vi "Common_GetClassAttrubutes.vi"(1 "Path(CtrlRenumf used if Path is empty)":path, 2 "CtlRefnum":refnum<vi>, 5 "error in (no error)":errorcluster, 6 "AttributeSerachP{atternNamesToIgnore":string[](array[string])) -> (12 "LibraryName":string, 15 "attributeInfo":T1[](array[typedef]), 19 "error out":errorcluster)   [LabVIEW 2020]
uses:
  CommonVIs_AttributeInfoType.ctl
  CommonVIs_AttributeDataType.ctl
  CommonVIs_VisibilityType.ctl
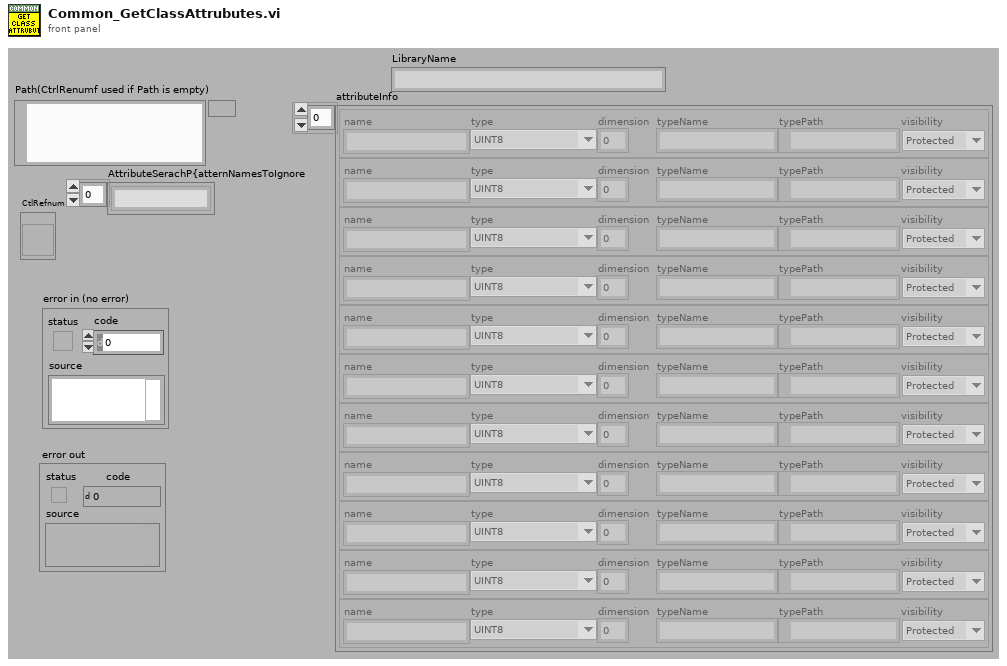
[diagram p1: front panel]
types:
  T1 = typedef "CommonVIs_AttributeInfoType.ctl" = cluster{"name":string, "type":T2, "dimension":i32, "typeName":string, "typePath":path, "visibility":T3}
  T2 = typedef "CommonVIs_AttributeDataType.ctl" = enum16{"UINT8", "INT8", "UINT16", "INT16", "UINT32", "INT32", "UINT64", "INT64", "SGL", "DBL", "EXT", "CSG", "CDB", "CXT", "TimeStamp", "STRING", "PATH", "BOOL", "ENUM", "RefNum", "VIRefNum", "LabVIEW Class", "Cluster", "Variant", "TypeDef", "Waveform", "LabVIEW Object", "Other", "void", "Set", "Map"}
  T3 = typedef "CommonVIs_VisibilityType.ctl" = enum16{"Public", "Private", "Protected"}
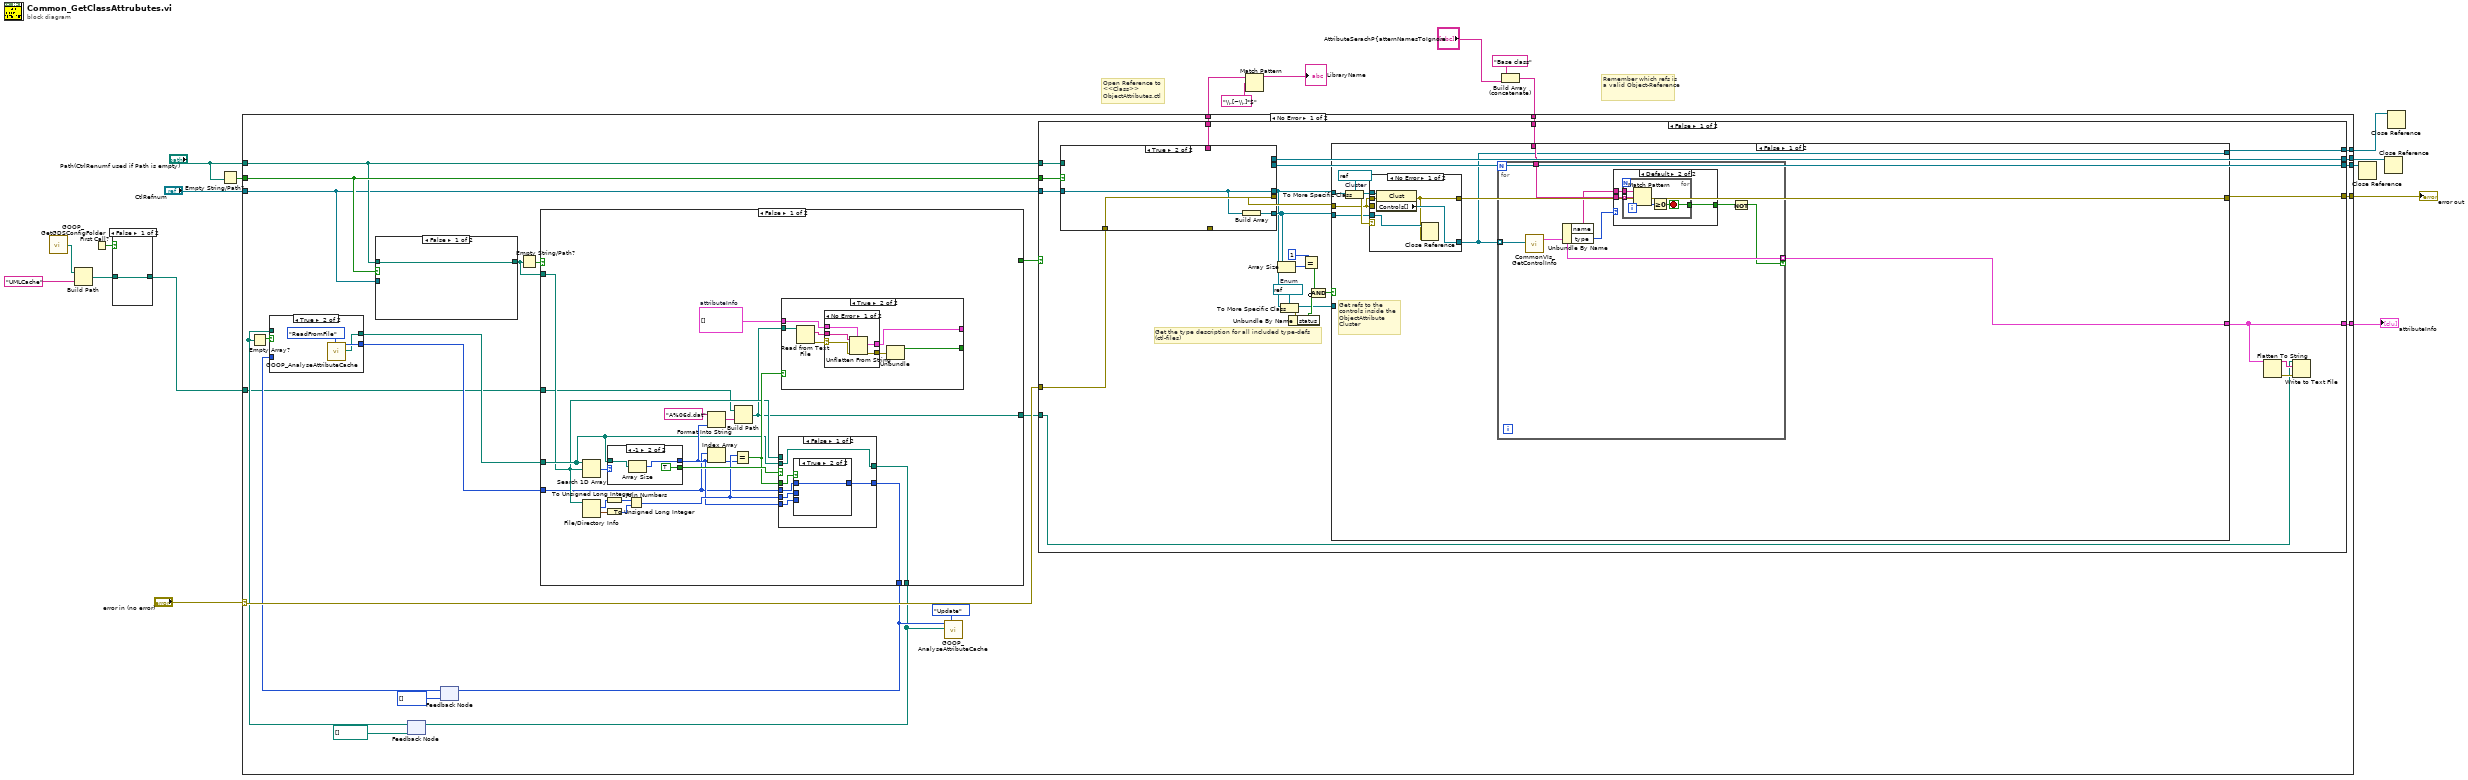
[diagram p0: block diagram]
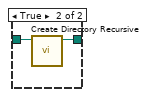
[diagram p2: hidden frame]
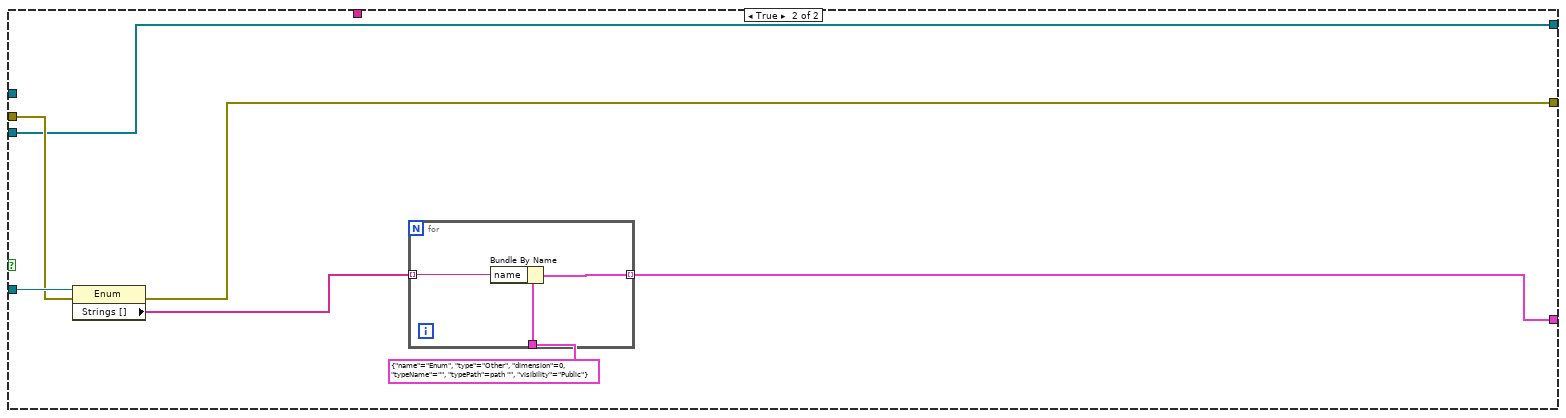
[diagram p6: hidden frame]
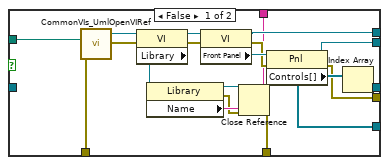
[diagram p7: hidden frame]
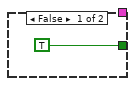
[diagram p9: hidden frame]
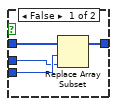
[diagram p11: hidden frame]
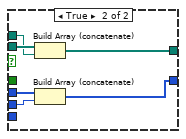
[diagram p12: hidden frame]
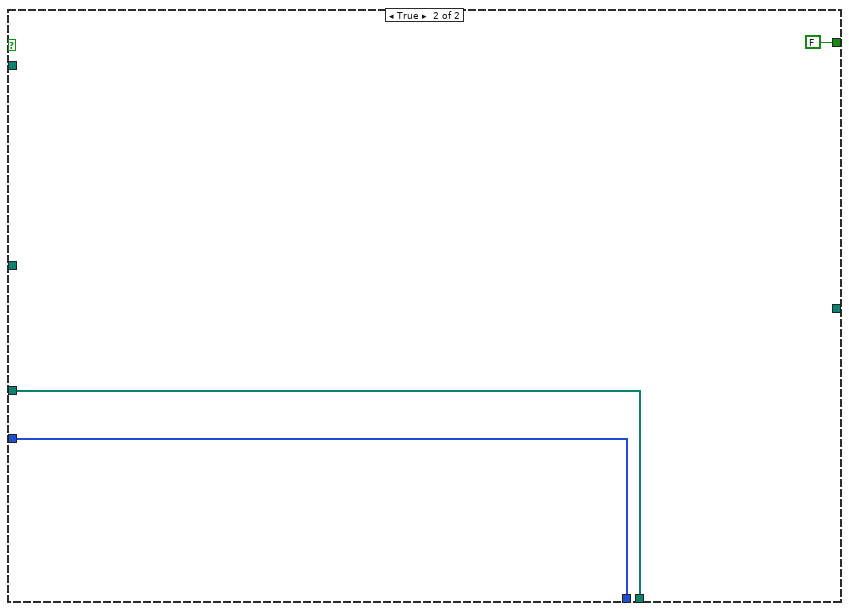
[diagram p14: hidden frame]
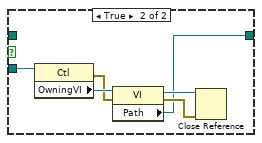
[diagram p15: hidden frame]
diagram:
  # "Remember which refs is a valid Object-Reference"
  # "Open Reference to <<Class>> ObjectAttributes.ctl"
  n1 = call "GOOP_GetGDSConfigFolder.vi"() -> ("GDSFolderPath"=w3:path)
  n2 = Build Path(base path=w3, name or relative path="UMLCache") -> (appended path=w6:path)
  n3 = First Call?() -> (First Call?: T/F=w5:bool)
  n4 = case shown="False" w5 {
    tunnel: w6 -> [w21 w23]
    tunnel: [w21 w22] -> w2
    frame False {
    }
    frame True {
      n5 = call <vilib>:"Create Directory Recursive.vi"("directory"=w23) -> ("directory copy"=w22:path)  [unwired: 4 in, 2 out]
    }
  }
  n6 = Empty String/Path?(string/path="Path(CtrlRenumf used if Path is empty)") -> (empty?=w13:bool)
  n7 = Build Array (concatenate)("Base class", "AttributeSerachP{atternNamesToIgnore") -> (w7:string[])
  n8 = case shown="No Error" "error in (no error)" {
    selector: "error in (no error)" -> [w43 w207]
    tunnel: [w49 _] -> w20
    tunnel: [w48 w207] -> w16
    tunnel: [w47 _] -> w19
    tunnel: w7 -> [w46 _]
    tunnel: [w45 _] -> w18
    tunnel: [w44 _] -> w17
    tunnel: "Path(CtrlRenumf used if Path is empty)" -> [w40 _]
    tunnel: w13 -> [w41 _]
    tunnel: "CtlRefnum" -> [w39 _]
    tunnel: [w42 _] -> w11
    tunnel: w2 -> [w28 _]
    frame No Error {
      n9 = case shown="False" w41 {
        tunnel: w40 -> [w200 _]
        tunnel: w39 -> [_ w206]
        tunnel: [w200 w201] -> w30
        frame False {
        }
        frame True {
          n10 = property class="Ctl"(reference=w206) -> (error out=w204:errorcluster, "OwningVI"=w205:refnum<vi>)  [unwired: 1 in, 1 out]
          n11 = property class="VI"(reference=w205, error in=w204) -> (reference out=w203:refnum<vi>, error out=w202:errorcluster, "Path"=w201:path)
          n12 = Close Reference(reference=w203, error in (no error)=w202) -> ()  [unwired: 1 out]
        }
      }
      n13 = feedback #1(path[] [] ("Paths")) -> (w33:path[])
      n14 = Empty Array?(array=w33) -> (empty?=w36:bool)
      n15 = feedback #2(u64[] [] ("Paths")) -> (w32:u64[])
      n16 = case shown="True" w36 {
        tunnel: [w50 w52] -> w31
        tunnel: w32 -> [w51 _]
        tunnel: [w51 w53] -> w29
        tunnel: w33 -> [w50 _]
        frame False {
        }
        frame True {
          n17 = call "GOOP_AnalyseAttributeCache.vi"("Actions"=enum16{"Update", "ReadFromFile", "SaveToFile"}."ReadFromFile") -> ("PathsOut"=w52:path[], "Date And Size ID(U64)Out"=w53:u64[])  [unwired: 8 in, 1 out]
        }
      }
      n18 = Empty String/Path?(string/path=w30) -> (empty?=w38:bool)
      n19 = case shown="False" w38 {
        tunnel: [_ FALSE] -> w37
        tunnel: w31 -> [w149 w197]
        tunnel: w30 -> [w148 _]
        tunnel: w29 -> [w147 w198]
        tunnel: w28 -> [w146 _]
        tunnel: [w145 w198] -> w26
        tunnel: [w144 w197] -> w25
        tunnel: [w142 _] -> w27
        frame False {
          w143 = T1[] []  # attributeInfo
          n20 = Search 1D Array(1D array=w149, element=w148) -> (index of element=w161:i32)  [unwired: 1 in]
          n21 = File/Directory Info(path=w148) -> (size=w158:i64, last mod=w159:timestamp)  [unwired: 1 in, 5 out]
          n22 = To Unsigned Long Integer(number=w158) -> (unsigned 32bit integer=w157:u32)
          n23 = To Unsigned Long Integer(number=w159) -> (unsigned 32bit integer=w156:u32)
          n24 = case shown="-1" w161 {
            selector: w161 -> [w193 _]
            tunnel: [_ TRUE] -> w160
            tunnel: [w193 w194] -> w150
            tunnel: w149 -> [_ w195]
            frame 0, Default {
            }
            frame -1 {
              n25 = Array Size(array=w195) -> (size(s)=w194:i32)
            }
          }
          n26 = Join Numbers(hi=w157, lo=w156) -> ((hi.lo)=w153:u64)
          n27 = Format Into String(format string="A%06d.dat", w150) -> (resulting string=w154:string)  [unwired: 2 in, 1 out]
          n28 = Index Array(array=w147, index=w150) -> (element=w152:u64)
          n29 = Equal?(x=w153, y=w152) -> (x = y?=w151:bool)
          n30 = Build Path(base path=w146, name or relative path=w154) -> (appended path=w142:path)
          n31 = case shown="False" w160 {
            tunnel: w149 -> [w181 w192]
            tunnel: [w181 w191] -> w144
            tunnel: w148 -> [_ w190]
            tunnel: w147 -> [w179 w187]
            tunnel: [w178 w188] -> w145
            tunnel: w153 -> [w176 w189]
            tunnel: w151 -> [w180 _]
            tunnel: w150 -> [w177 _]
            frame False {
              n32 = case shown="True" w180 {
                tunnel: w179 -> [w185 w186]
                tunnel: [w184 w186] -> w178
                tunnel: w177 -> [w183 _]
                tunnel: w176 -> [w182 _]
                frame False {
                  n33 = Replace Array Subset(array=w185, new element=w182, index=w183) -> (w184:u64[])
                }
                frame True {
                }
              }
            }
            frame True {
              n34 = Build Array (concatenate)(w192, w190) -> (w191:path[])
              n35 = Build Array (concatenate)(w187, w189) -> (w188:u64[])
            }
          }
          n36 = case shown="True" w151 {
            tunnel: [TRUE ("status") w163] -> _
            tunnel: w143 -> [_ w167]
            tunnel: [_ w166] -> _
            tunnel: w142 -> [_ w165]
            frame False {
            }
            frame True {
              n37 = Read from Text File(file (use dialog)=w165) -> (text=w168:string, error out=w169:errorcluster)  [unwired: 3 in, 2 out]
              n38 = case shown="No Error" w169 {
                selector: w169 -> [w174 w175]
                tunnel: [w173 w175] -> w164
                tunnel: w168 -> [w172 _]
                tunnel: w167 -> [w171 _]
                tunnel: [w170 _] -> w166
                frame No Error {
                  n39 = Unflatten From String(type=w171, binary string=w172, error in (no error)=w174) -> (value=w170:T1[], error out=w173:errorcluster)  [unwired: 2 in, 1 out]
                }
                frame Error {
                }
              }
              n40 = Unbundle(w164) -> ("status"=w163:bool)  [unwired: 2 out]
            }
          }
        }
        frame True {
        }
      }
      n41 = feedback-in #1(w25) -> ()
      n42 = feedback-in #2(w26) -> ()
      n43 = call "GOOP_AnalyseAttributeCache.vi"("Actions"=enum16{"Update", "ReadFromFile", "SaveToFile"}."Update", "Paths"=w25, "Date And Size ID(U64)"=w26) -> ()  [unwired: 6 in, 3 out]
      n44 = case shown="False" w37 {
        tunnel: [w79 _] -> w49
        tunnel: [w78 _] -> w48
        tunnel: [w56 _] -> w47
        tunnel: w46 -> [w77 _]
        tunnel: [w76 _] -> w45
        tunnel: [w74 _] -> w44
        tunnel: w43 -> [w73 _]
        tunnel: [w62 _] -> w42
        tunnel: w41 -> [w61 _]
        tunnel: w40 -> [w60 _]
        tunnel: w39 -> [w59 _]
        tunnel: w27 -> [w55 _]
        frame False {
          w71 = refnum<vi> refnum  # Enum
          # "Get the type description for all included type-defs (ctl-files)"
          n45 = case shown="True" w61 {
            tunnel: [w135 w140] -> w70
            tunnel: [w133 _] -> w79
            tunnel: [w132 _] -> w76
            tunnel: [w131 w139] -> w72
            tunnel: [w130 w141] -> w75
            tunnel: w73 -> [w124 w141]
            tunnel: w60 -> [w127 _]
            tunnel: w59 -> [_ w140]
            tunnel: [w128 _] -> w62
            tunnel: [w121 _] -> _
            frame False {
              n46 = call "CommonVIs_UmlOpenVIRef.vi"("error in"=w124, "ViPath/ViName"=w127) -> ("error out"=w126:errorcluster, "vi reference"=w125:refnum<vi>)  [unwired: 2 in, 6 out]
              n47 = property class="VI"(reference=w125, error in=w126) -> (reference out=w138:refnum<vi>, error out=w137:errorcluster, "Library"=w129:refnum<vi>)
              n48 = property class="Library"(reference=w129) -> (reference out=w123:refnum<vi>, error out=w122:errorcluster, "Name"=w128:string)  [unwired: 1 in]
              n49 = property class="VI"(reference=w138, error in=w137) -> (reference out=w133:refnum<vi>, error out=w134:errorcluster, "Front Panel"=w136:refnum<vi>)
              n50 = Close Reference(reference=w123, error in (no error)=w122) -> (error out=w121:errorcluster)
              n51 = property class="Pnl"(reference=w136, error in=w134) -> (reference out=w132:refnum<vi>, error out=w130:errorcluster, "Controls[]"=w131:refnum<vi>[])
              n52 = Index Array(array=w131) -> (element=w135:refnum<vi>)  [unwired: 1 in]
            }
            frame True {
              n53 = Build Array(w140) -> (w139:refnum<vi>[])
            }
          }
          n54 = Array Size(array=w72) -> (size(s)=w68:i32)
          n55 = To More Specific Class(target class=w71, reference=w70) -> (specific class reference=w63:refnum<vi>, error out=w69:errorcluster)  [unwired: 1 in]
          n56 = Unbundle By Name(w69) -> ("status"=w66:bool)
          n57 = Equal?(x=1, y=w68) -> (x = y?=w65:bool)
          n58 = Compound Arithmetic op=AND(w65, invert w66) -> (w64:bool)
          n59 = case shown="False" w64 {
            tunnel: [w87 w113] -> w78
            tunnel: [w86 w114] -> w56
            tunnel: w77 -> [w85 _]
            tunnel: w75 -> [w83 w112]
            tunnel: [w82 w111] -> w74
            tunnel: w72 -> [w81 w111]
            tunnel: w70 -> [w80 _]
            tunnel: w63 -> [_ w117]
            frame False {
              w89 = refnum<vi> refnum  # Cluster
              # "Get refs to the controls inside the ObjectAttribute Cluster"
              n60 = To More Specific Class(target class=w89, reference=w80) -> (specific class reference=w88:refnum<vi>, error out=w84:errorcluster)  [unwired: 1 in]
              n61 = case shown="No Error" w84 {
                tunnel: w88 -> [w108 _]
                tunnel: [w106 w109] -> w82
                tunnel: w83 -> [w107 _]
                tunnel: [w104 w110] -> w87
                tunnel: w81 -> [w105 w109]
                tunnel: w83 -> [_ w110]
                frame No Error {
                  n62 = property class="Clust"(reference=w108, error in=w107) -> (error out=w104:errorcluster, "Controls[]"=w106:refnum<vi>[])  [unwired: 1 out]
                  n63 = Close Reference(reference=w105, error in (no error)=w104) -> ()  [unwired: 1 out]
                }
                frame Error {
                }
              }
              n64 = for {
                tunnel: w82 -> [w96] mode=indexing
                tunnel: w85 -> [w94]
                tunnel: [w91] -> w86 mode=indexing if=w90
                n65 = call "CommonVIs_GetControlInfo.vi"("CtlRefnum"=w96) -> ("attributeInfoType"=w91:T1)  [unwired: 17 in, 1 out]
                n66 = Unbundle By Name(w91) -> ("name"=w93:string, "type"=w95:T2)
                n67 = case shown="Default" w95 {
                  tunnel: [_ w97] -> w92
                  tunnel: w94 -> [_ w99]
                  tunnel: w93 -> [_ w98]
                  frame "LabVIEW Class" {
                  }
                  frame Default {
                    n68 = for {
                      tunnel: w98 -> [w102]
                      tunnel: w99 -> [w101] mode=indexing
                      tunnel: [w100] -> w97
                      stop <- w100 stop-if-true
                      n69 = Match Pattern(string=w102, regular expression=w101) -> (offset past match=w103:i32)  [unwired: 4 out]
                      n70 = Greater Or Equal To 0?(x=w103) -> (x >= 0?=w100:bool)
                    }
                  }
                }
                n71 = Not(x=w92) -> (.not. x?=w90:bool)
              }
            }
            frame True {
              n72 = property class="Enum"(reference=w117, error in=w112) -> (error out=w113:errorcluster, "Strings []"=w115:string[])  [unwired: 1 out]
              n73 = for {
                tunnel: T1 {"name"="Enum", "type"=enum."Other", "dimension"=0, "typeName"="", "typePath"=path "", "visibility"=enum."Public"} ("attributeInfoType") -> [w120]
                tunnel: w115 -> [w119] mode=indexing
                tunnel: [w118] -> w114 mode=indexing
                n74 = Bundle By Name(cluster=w120, "name"=w119) -> (w118:T1)
              }
            }
          }
          n75 = Flatten To String(anything=w56) -> (data string=w57:string, error out=w58:errorcluster)  [unwired: 3 in, 1 out]
          n76 = Write to Text File(file (use dialog)=w55, text=w57, error in=w58) -> ()  [unwired: 1 in, 3 out]
        }
        frame True {
        }
      }
    }
    frame Error {
    }
  }
  "error out" <- w16
  "attributeInfo" <- w19
  n77 = Match Pattern(string=w11, regular expression="\\.[~\\.]*$") -> (before substring=→"LibraryName":string)  [unwired: 4 out]
  n78 = Close Reference(reference=w18) -> ()  [unwired: 1 in, 1 out]
  n79 = Close Reference(reference=w20) -> ()  [unwired: 1 in, 1 out]
  n80 = Close Reference(reference=w17) -> ()  [unwired: 1 in, 1 out]
